vi "Configure Offset and Limits (Power Meter).vi"(0 "VISA resource name":refnum<visa-resource-name>, 1 "Offset (0 dBm)":dbl, 2 "Upper Limit Value (100 dBm)":dbl=100.0, 5 "Enable Reference Power (F: Disable)":bool, 7 "Reference Power (0 dBm)":dbl, 9 "Enable Offset (F: Disable)":bool, 11 "error in (no error)":errorcluster, 12 "Enable Limit (F: Disable)":bool, 13 "Lower Limit Value (-100 dBm)":dbl=-100.0) -> (4 "VISA resource name out":refnum<visa-resource-name>, 15 "error out":errorcluster)   [LabVIEW 2022 SP3, in "Agilent N934X Series.lvlib"]
doc: "Configures the general setting for offset and limits of Power Meter Option.\n\nNote:\nThis VI is only applicable for N9321C, N9322C, N9323C, N9324C models."
uses:
  <instrlib>/Agilent N934X Series/Agilent N934X Series.lvlib
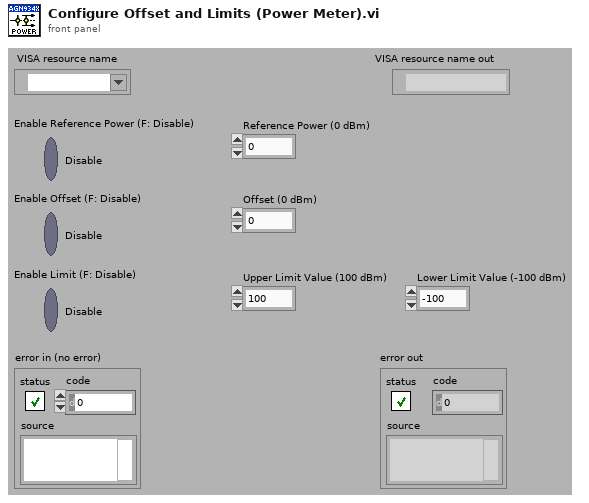
[diagram p1: front panel]
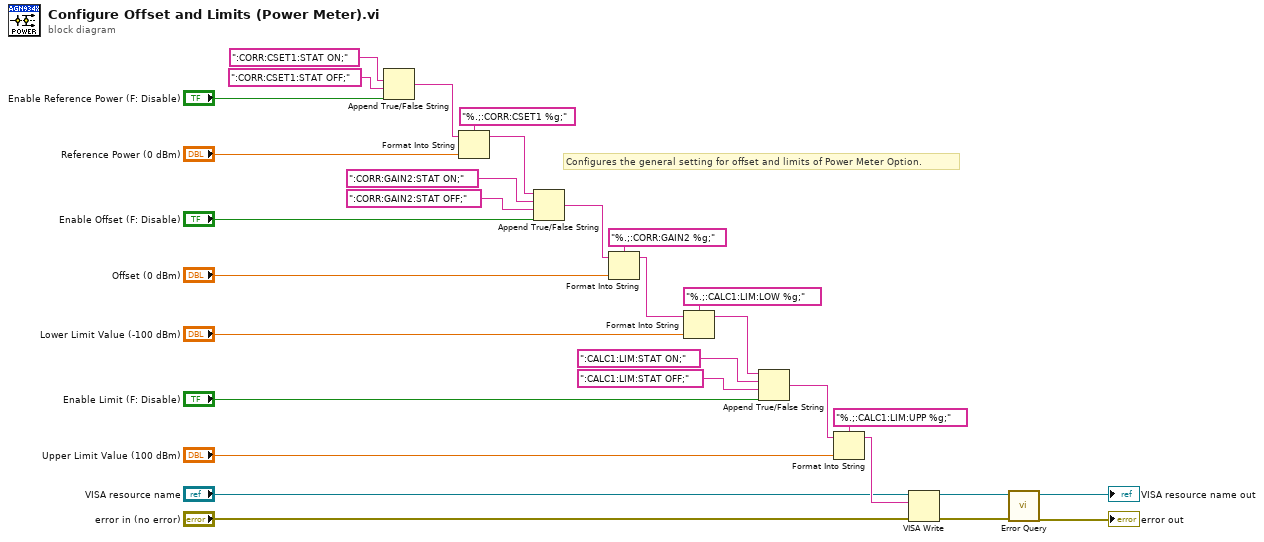
[diagram p0: block diagram]
diagram:
  # "Configures the general setting for offset and limits of Power Meter Option."
  n1 = Append True/False String(1:"Enable Reference Power (F: Disable)", 2:":CORR:CSET1:STAT OFF;", 3:":CORR:CSET1:STAT ON;") -> (0:w27:string)  [unwired: 1 in]
  n2 = Format Into String(format string="%.;:CORR:CSET1 %g;", initial string=w27, "Reference Power (0 dBm)") -> (resulting string=w24:string)  [unwired: 1 in, 1 out]
  n3 = Append True/False String(1:"Enable Offset (F: Disable)", 2:":CORR:GAIN2:STAT OFF;", 3:":CORR:GAIN2:STAT ON;", 4:w24) -> (0:w20:string)
  n4 = Format Into String(format string="%.;:CORR:GAIN2 %g;", initial string=w20, "Offset (0 dBm)") -> (resulting string=w17:string)  [unwired: 1 in, 1 out]
  n5 = Format Into String(format string="%.;:CALC1:LIM:LOW %g;", initial string=w17, "Lower Limit Value (-100 dBm)") -> (resulting string=w14:string)  [unwired: 1 in, 1 out]
  n6 = Append True/False String(1:"Enable Limit (F: Disable)", 2:":CALC1:LIM:STAT OFF;", 3:":CALC1:LIM:STAT ON;", 4:w14) -> (0:w10:string)
  n7 = Format Into String(format string="%.;:CALC1:LIM:UPP %g;", initial string=w10, "Upper Limit Value (100 dBm)") -> (resulting string=w7:string)  [unwired: 1 in, 1 out]
  n8 = VISA Write(VISA resource name="VISA resource name", write buffer=w7, error in (no error)="error in (no error)") -> (VISA resource name out=w4:refnum<visa-resource-name>, error out=w3:errorcluster)  [unwired: 1 out]
  n9 = call <instrlib>:"Error Query.vi"("error in (no error)"=w3, "VISA resource name"=w4) -> ("error out"=→"error out":errorcluster, "VISA resource name out"=→"VISA resource name out":refnum<visa-resource-name>)  [unwired: 6 in, 2 out]
